vi "Periodic Tasks.vi"(8 "error out 2":errorcluster) -> ()   [LabVIEW 2012]
doc: "This VI runs in parallel to other tasks. It can contain as many user-defined periodic loops as you need. These can carry out PID or other sorts of timed response."
panel:
  in  "milliseconds to wait":u32
  out "Average Difference":dbl
  out "RPM":dbl
  out "Stopped":bool
  out "Period (sec)":dbl
  out "error out":errorcluster
  out "Direction":bool
  out "Value":i32
  in  "Motor Control":dbl
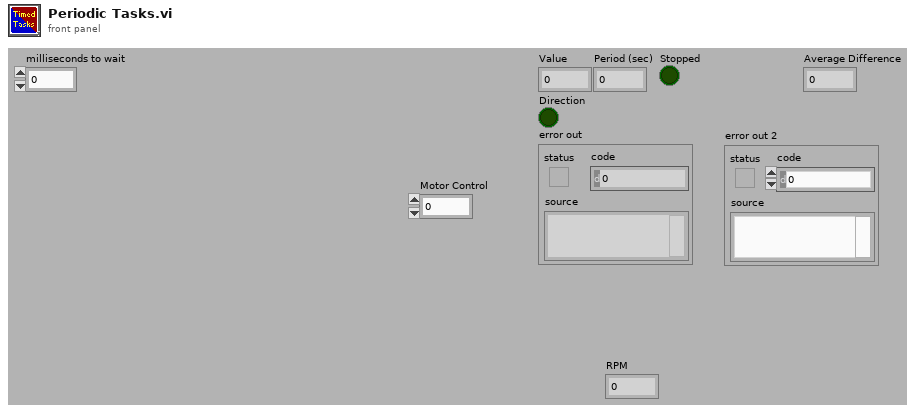
[diagram p1: front panel]
types:
  T1 = typedef "WPI_CounterDevRef.ctl" = cluster{"DevStatus":errorcluster, "CntIndex":T2}
  T2 = typedef "FPGA_CounterCtrSystemIndex.ctl" = enum8{"Ctr 0", "Ctr 1", "Ctr 2", "Ctr 3", "Ctr 4", "Ctr 5", "Ctr 6", "Ctr 7", "Invalid"}
  T3 = typedef "WPI_MotorControlDeviceRef.ctl" = cluster{"DeviceStatus":errorcluster, "Type":enum16{"PWM", "CAN"}, "PWM":cluster{"Digital Module":T4, "PWM Channel":T5, "DeadBand":T6}, "CAN":cluster{"Device Number":u8, "Control Mode":T7, "Semaphore":T8, "Max Vout":dbl}, "Invert":bool, "TransformRef":T9, "InvTransformRef":T9}
  T4 = typedef "FPGA_TypedefDigitalModule.ctl" = enum16{"Digital Module 1", "Digital Module 2"}
  T5 = typedef "FPGA_DIOPWMChannel.ctl" = enum8{"PWM 1", "PWM 2", "PWM 3", "PWM 4", "PWM 5", "PWM 6", "PWM 7", "PWM 8", "PWM 9", "PWM 10", "Invalid"}
  T6 = typedef "WPI_PWMDeadband.ctl" = cluster{"Name":string, "maxPositivePwm":i32, "minPositivePwm":i32, "centerPwm":i32, "maxNegativePwm":i32, "minNegativePwm":i32, "angularRange":u16}
  T7 = typedef "WPI_CANJaguar_ControlMode.ctl" = enum8{"Percent VBus", "Current", "Speed", "Position", "Voltage"}
  T8 = typedef "Semaphore RefNum" = refnum<k1>
  T9 = typedef "WPI_PWMTransform_ConPane.ctl" = refnum<vi>
  T10 = cluster{"[0]":dbl, "[1]":dbl, "[2]":dbl, "[3]":dbl, "[4]":dbl, "[5]":dbl, "[6]":dbl, "[7]":dbl, "[8]":dbl}
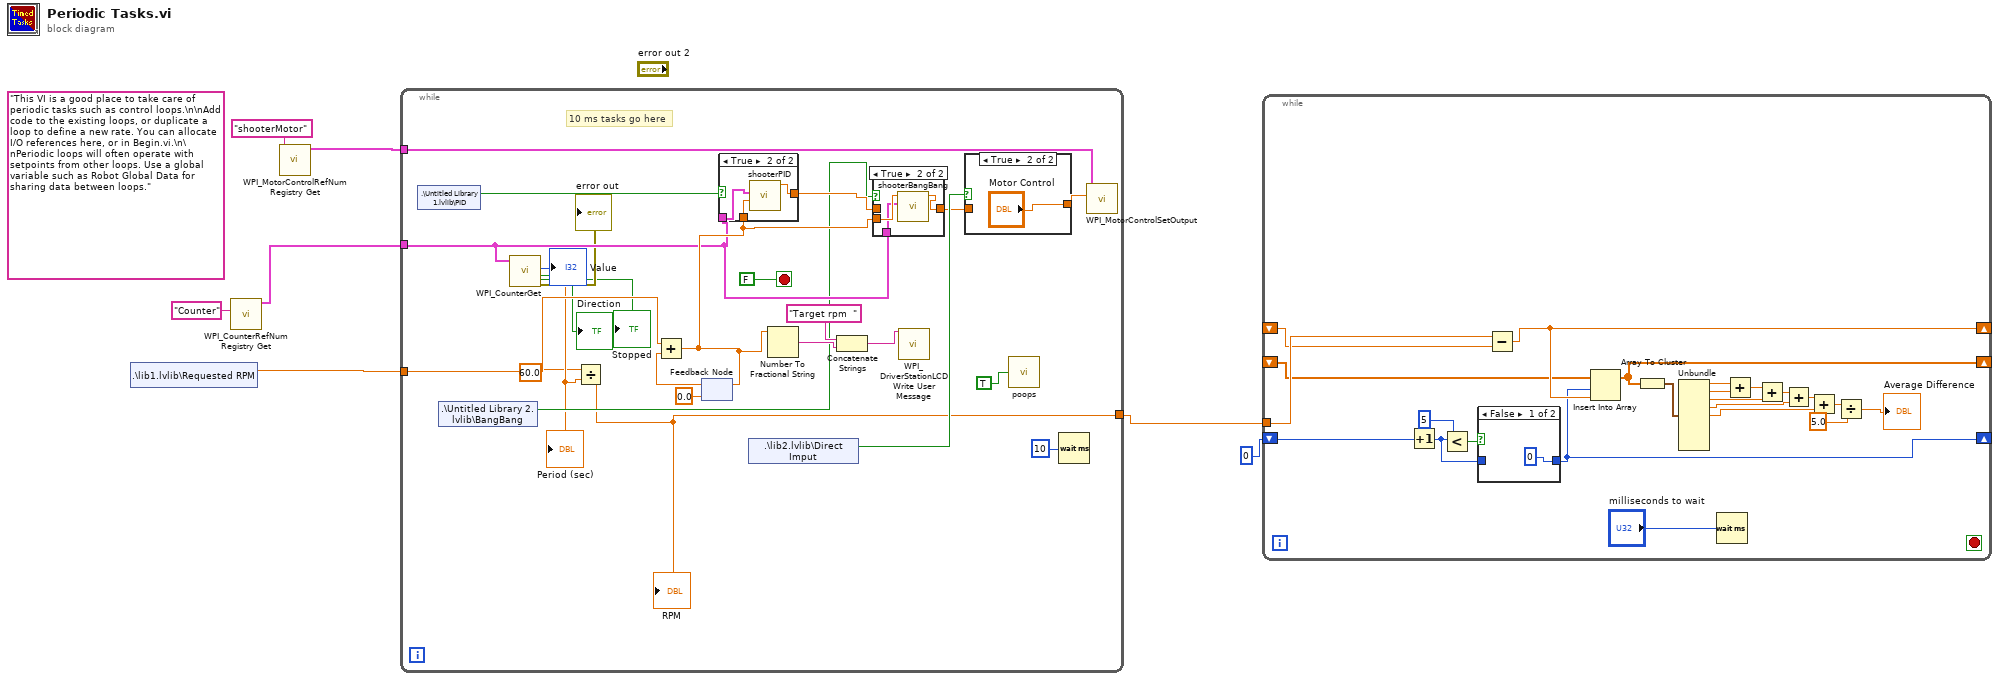
[diagram p0: block diagram]
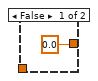
[diagram p5: hidden frame]
diagram:
  (unwired) "This VI is a good place to take care of periodic tasks such as control loops.\n\nAdd code to the existing loops, or duplicate a loop to define a new rate. You can allocate I/O references here, or in Begin.vi.\n\nPeriodic loops will often operate with setpoints from other loops. Use a global variable such as Robot Global Data for sharing data between loops."
  n1 = shared-variable ".\\lib1.lvlib\\Requested RPM"() -> (w3:dbl)  [unwired: 1 in, 1 out]
  n2 = call <vilib>:"WPI_CounterRefNum Registry Get.vi"("refnum name"="Counter") -> ("CounterDevRef"=w7:T1)  [unwired: 9 in, 1 out]
  n3 = call <vilib>:"WPI_MotorControlRefNum Registry Get.vi"("refnum name"="shooterMotor") -> ("MotorControlDevRef"=w6:T3)  [unwired: 9 in, 1 out]
  n4 = while {
    tunnel: w7 -> [w16]
    tunnel: w6 -> [w29]
    tunnel: w3 -> [w28]
    tunnel: [w8] -> w2
    stop <- FALSE stop-if-true
    # "10 ms tasks go here"
    n5 = shared-variable ".\\Untitled Library 1.lvlib\\PID"() -> (w30:bool)  [unwired: 1 in, 1 out]
    n6 = shared-variable ".\\Untitled Library 2.lvlib\\BangBang"() -> (w11:bool)  [unwired: 1 in, 1 out]
    n7 = call <vilib>:"WPI_CounterGet.vi"("CounterDevRef in"=w16) -> ("error out"=→"error out":errorcluster, "Direction"=→"Direction":bool, "Value"=→"Value":i32, "Period (sec)"=w10:dbl, "Stopped"=→"Stopped":bool)  [unwired: 5 in, 1 out]
    "Period (sec)" <- w10
    n8 = Divide(x=60.0, y=w10) -> (x/y=w8:dbl)
    "RPM" <- w8
    n9 = feedback #1(0.0) -> (w27:dbl)
    n10 = Add(x=w28, y=w27) -> (x+y=w21:dbl)
    n11 = feedback-in #1(w21) -> ()
    n12 = case shown="True" w30 {
      tunnel: w16 -> [_ w42]
      tunnel: [0.0 w41] -> w25
      tunnel: w21 -> [_ w40]
      frame False {
      }
      frame True {
        n13 = call "shooterPID.vi"("rpmTarget"=w40, "CounterDevRef"=w42) -> ("output"=w41:dbl)  [unwired: 9 in]
      }
    }
    n14 = shared-variable ".\\lib2.lvlib\\Direct Imput"() -> (w24:bool)  [unwired: 1 in, 1 out]
    n15 = Number To Fractional String(number=w21) -> (F-format string=w20:string)  [unwired: 3 in]
    n16 = Concatenate Strings("Target rpm  " ("string"), w20) -> (w18:string)
    n17 = case shown="True" w11 {
      tunnel: w25 -> [w35 _]
      tunnel: [w35 w38] -> w23
      tunnel: w21 -> [_ w37]
      tunnel: w16 -> [_ w36]
      frame False {
      }
      frame True {
        n18 = call "shooterBangBang.vi"("CounterDevRef in"=w36, "rpmTarget"=w37) -> ("Output"=w38:dbl)  [unwired: 9 in]
      }
    }
    n19 = call <vilib>:"WPI_DriverStationLCDWrite User Message.vi"("line text"=w18) -> ()  [unwired: 14 in, 1 out]
    n20 = case shown="True" w24 {
      tunnel: w23 -> [w33 _]
      tunnel: [w33 "Motor Control"] -> w22
      frame False {
      }
      frame True {
      }
    }
    n21 = call "poops.vi"("enabled?"=TRUE) -> ()  [unwired: 2 in]
    n22 = Wait (ms)(milliseconds to wait=u32 10) -> ()  [unwired: 1 out]
    n23 = call <vilib>:"WPI_MotorControlSetOutput.vi"("Output"=w22, "MotorControlDevRef"=w29) -> ()  [unwired: 7 in, 3 out]
  }
  n24 = while {
    tunnel: w2 -> [w65]
    shift-right: [w63] -> _
    shift-left: _ -> [w64]
    shift-right: [w58] -> _
    shift-left: _ -> [w62]
    shift-right: [w50] -> _
    shift-left: 0 -> [w49]
    stop <- _ stop-if-true
    n25 = Increment(x=w49) -> (x+1=w59:i32)
    n26 = Less?(x=w59, y=5) -> (x < y?=w60:bool)
    n27 = case shown="False" w60 {
      tunnel: w59 -> [_ w67]
      tunnel: [0 w67] -> w50
      frame False {
      }
      frame True {
      }
    }
    n28 = Subtract(x=w65, y=w64) -> (x-y=w63:dbl)
    n29 = Insert Into Array(array=w62, index=w50, new element=w63) -> (w58:dbl[])
    n30 = Array To Cluster(array=w58) -> (cluster=w57:T10)
    n31 = Unbundle(w57) -> ("[0]"=w55:dbl, "[1]"=w56:dbl, "[2]"=w53:dbl, "[3]"=w51:dbl, "[4]"=w47:dbl)  [unwired: 4 out]
    n32 = Wait (ms)(milliseconds to wait="milliseconds to wait") -> ()  [unwired: 1 out]
    n33 = Add(x=w55, y=w56) -> (x+y=w54:dbl)
    n34 = Add(x=w54, y=w53) -> (x+y=w52:dbl)
    n35 = Add(x=w52, y=w51) -> (x+y=w48:dbl)
    n36 = Add(x=w48, y=w47) -> (x+y=w46:dbl)
    n37 = Divide(x=w46, y=5.0) -> (x/y=→"Average Difference":dbl)
  }
